vi "IMAQ Convert From OCR Read Report Internal 2.vi"(1 "Character Reports (internal)":T2(array[cluster]) {"Character Statistics"."Threshold Range"."Upper value" format="%.2f"; "Character Statistics"."Threshold Range"."Lower value" format="%.2f"}) -> (0 "Character Reports":T1[](array[typedef]) {"Character Statistics"."Threshold Range"."Upper value" format="%.2f"; "Character Statistics"."Threshold Range"."Lower value" format="%.2f"})   [LabVIEW 2020]
uses:
  IMAQ OCR Character Report 2.ctl
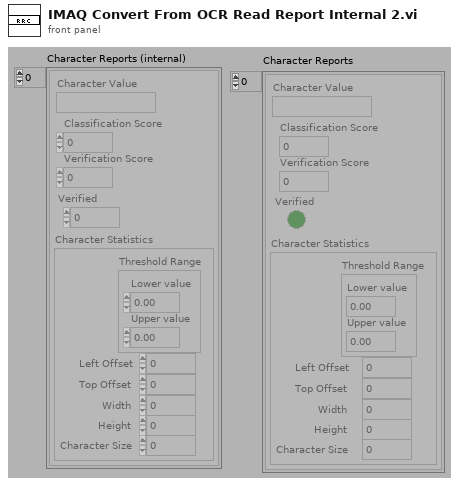
[diagram p1: front panel]
types:
  T1 = typedef "IMAQ OCR Character Report 2.ctl" = cluster{"Character Value":string, "Classification Score":i32, "Verification Score":i32, "Verified":bool, "Character Statistics":cluster{"Threshold Range":cluster{"Lower value":sgl, "Upper value":sgl}, "Left Offset":i32, "Top Offset":i32, "Width":i32, "Height":i32, "Character Size":i32}}
  T2 = cluster{"Character Value":string, "Classification Score":i32, "Verification Score":i32, "Verified":i32, "Character Statistics":cluster{"Threshold Range":cluster{"Lower value":sgl, "Upper value":sgl}, "Left Offset":i32, "Top Offset":i32, "Width":i32, "Height":i32, "Character Size":i32}}[]
  T3 = cluster{"Threshold Range":cluster{"Lower value":sgl, "Upper value":sgl}, "Left Offset":i32, "Top Offset":i32, "Width":i32, "Height":i32, "Character Size":i32}
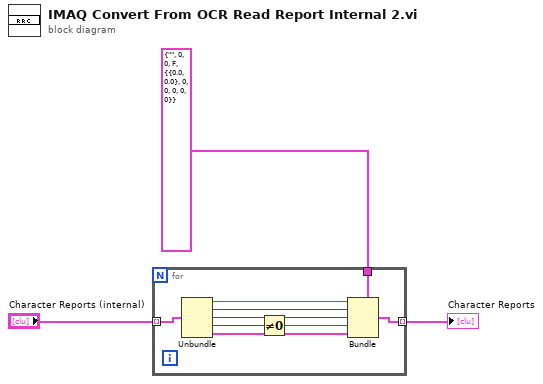
[diagram p0: block diagram]
diagram:
  n1 = for {
    tunnel: "Character Reports (internal)" -> [w12] mode=indexing
    tunnel: [w7] -> w2 mode=indexing
    tunnel: T1 {"Character Value"="", "Classification Score"=0, "Verification Score"=0, "Verified"=FALSE, "Character Statistics"={"Threshold Range"={"Lower value"=0.0, "Upper value"=0.0}, "Left Offset"=0, "Top Offset"=0, "Width"=0, "Height"=0, "Character Size"=0}} ("Character Report") -> [w4]
    n2 = Unbundle(w12) -> ("Character Value"=w11:string, "Classification Score"=w10:i32, "Verification Score"=w9:i32, "Verified"=w8:i32, "Character Statistics"=w6:T3)
    n3 = Not Equal To 0?(x=w8) -> (x != 0?=w5:bool)
    n4 = Bundle(cluster=w4, "Character Value"=w11, "Classification Score"=w10, "Verification Score"=w9, "Verified"=w5, "Character Statistics"=w6) -> (w7:T1)
  }
  "Character Reports" <- w2
